vi "基础6.vi"() -> ()   [LabVIEW 2014]
panel:
  out "灯":bool
  in  "报警":dbl(slide) scale=0.0..100.0
  out "温度计":dbl(slide) scale=0.0..100.0
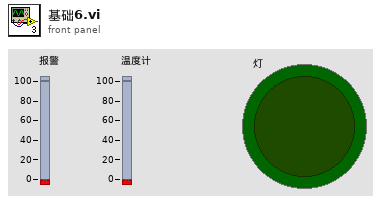
[diagram p1: front panel]
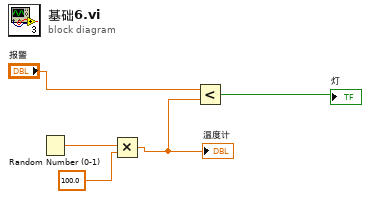
[diagram p0: block diagram]
diagram:
  n1 = Random Number (0-1)() -> (number: 0 to 1=w5:dbl)
  n2 = Multiply(x=w5, y=100.0) -> (x*y=w2:dbl)
  "温度计" <- w2
  n3 = Less?(x="报警", y=w2) -> (x < y?=→"灯":bool)
